vi "Initialize.vi"(0 "DMA FIFO":refnum<k21>="DataSGL7", 5 "instance":u8) -> (4 "subsystem":refnum<class "Single Address Space Collection.lvclass">, 6 "AddressSpace":refnum<class "WaveformAddressSpace.lvclass">)   [LabVIEW 2017, in "WaveformAddressSpace.lvclass"]
uses:
  WaveformAddressSpace.lvclass
  C:/Program Files (x86)/National Instruments/LabVIEW 2017/instr.lib/_niInstr/Instruction Framework/v1/FPGA/Interfaces/Address Space/Address Space.lvclass
  <instrlib>/_niInstr/Instruction Framework/v1/FPGA/Helper Classes/Single Address Space Collection/Single Address Space Collection.lvclass
  Registers.ctl
  WaveformAddressSpace.lvclass/WaveformAddressSpace.ctl
  <vilib>/rvi/DataTransferAndStorage/Container/Common/niFpgaContainerGetUniqueNameForEmu.vi
  <vilib>/rvi/DataTransferAndStorage/Container/Common/niFpgaContainerSetEmuInfo.vi
  <vilib>/rvi/eio/common/nirviEmuReportErrorAndStop.vi
  <vilib>/rvi/LocalResourceManager/LocalResourceManager.xnode
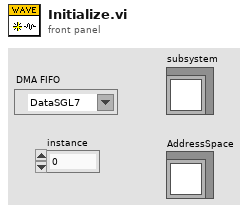
[diagram p1: front panel]
types:
  T1 = typedef "WaveformAddressSpace.lvclass/Registers.ctl" = cluster{"oclk_freq":refnum<k21>, "data_rate":refnum<k21>, "oclk_div":refnum<k21>, "oclk_mult":refnum<k21>, "AcquisitionType":refnum<k21>, "SamplesPerChan":refnum<k21>, "NumberOfChannels":refnum<k21>, "stop":refnum<k21>, "FIFO":refnum<k21>, "FirstRead":refnum<k21>, "ErrorCode":refnum<k21>, "ChannelCount":refnum<k21>, "Finished":refnum<k21>, "DMA_FIFO_Full":refnum<k21>, "ModuleUnderflow":refnum<k21>, "ConfigReadyIRQ":refnum<k21>, "ConfigReadyAck":refnum<k21>, "SynchStartIRQ":refnum<k21>, "SynchStartAck":refnum<k21>, "UnderflowCount":refnum<k21>, "FirstReadReset":refnum<k21>}
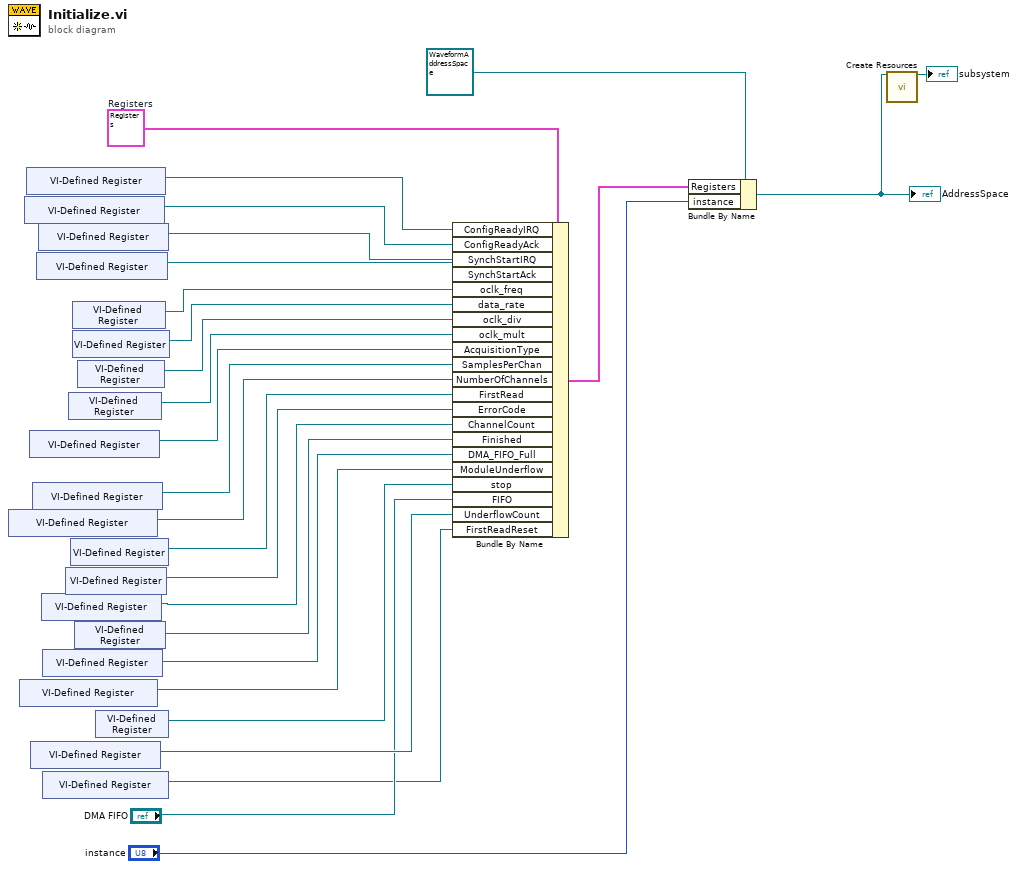
[diagram p0: block diagram]
diagram:
  w12 = T1 {"oclk_freq"="", "data_rate"="", "oclk_div"="", "oclk_mult"="", "AcquisitionType"="", "SamplesPerChan"="", "NumberOfChannels"="", "stop"="", "FIFO"="", "FirstRead"="", "ErrorCode"="", "ChannelCount"="", "Finished"="", "DMA_FIFO_Full"="", "ModuleUnderflow"="", "ConfigReadyIRQ"="Register", "ConfigReadyAck"="Register", "SynchStartIRQ"="Register", "SynchStartAck"="Register", "UnderflowCount"="", "FirstReadReset"="Register"}  # Registers
  n1 = xnode "VI-Defined Register"() -> ("Register Out"=w21:refnum<k21>)
  n2 = xnode "VI-Defined Register"() -> ("Register Out"=w13:refnum<k21>)
  n3 = xnode "VI-Defined Register"() -> ("Register Out"=w7:refnum<k21>)
  n4 = xnode "VI-Defined Register"() -> ("Register Out"=w8:refnum<k21>)
  n5 = xnode "VI-Defined Register"() -> ("Register Out"=w23:refnum<k21>)
  n6 = xnode "VI-Defined Register"() -> ("Register Out"=w4:refnum<k21>)
  n7 = xnode "VI-Defined Register"() -> ("Register Out"=w22:refnum<k21>)
  n8 = xnode "VI-Defined Register"() -> ("Register Out"=w5:refnum<k21>)
  n9 = xnode "VI-Defined Register"() -> ("Register Out"=w6:refnum<k21>)
  n10 = xnode "VI-Defined Register"() -> ("Register Out"=w16:refnum<k21>)
  n11 = xnode "VI-Defined Register"() -> ("Register Out"=w14:refnum<k21>)
  n12 = xnode "VI-Defined Register"() -> ("Register Out"=w1:refnum<k21>)
  n13 = xnode "VI-Defined Register"() -> ("Register Out"=w17:refnum<k21>)
  n14 = xnode "VI-Defined Register"() -> ("Register Out"=w24:refnum<k21>)
  n15 = xnode "VI-Defined Register"() -> ("Register Out"=w19:refnum<k21>)
  n16 = xnode "VI-Defined Register"() -> ("Register Out"=w18:refnum<k21>)
  n17 = xnode "VI-Defined Register"() -> ("Register Out"=w26:refnum<k21>)
  n18 = xnode "VI-Defined Register"() -> ("Register Out"=w15:refnum<k21>)
  n19 = xnode "VI-Defined Register"() -> ("Register Out"=w25:refnum<k21>)
  n20 = xnode "VI-Defined Register"() -> ("Register Out"=w20:refnum<k21>)
  n21 = Bundle By Name(cluster=w12, "ConfigReadyIRQ"=w8, "ConfigReadyAck"=w7, "SynchStartIRQ"=w6, "SynchStartAck"=w5, "oclk_freq"=w18, "data_rate"=w26, "oclk_div"=w25, "oclk_mult"=w24, "AcquisitionType"=w23, "SamplesPerChan"=w22, "NumberOfChannels"=w21, "FirstRead"=w19, "ErrorCode"=w17, "ChannelCount"=w16, "Finished"=w15, "DMA_FIFO_Full"=w14, "ModuleUnderflow"=w13, "stop"=w20, "FIFO"="DMA FIFO", "UnderflowCount"=w4, "FirstReadReset"=w1) -> (w11:T1)
  n22 = Bundle By Name(cluster=refnum<class "WaveformAddressSpace.lvclass"> refnum ("WaveformAddressSpace.lvclass"), "Registers"=w11, "instance"="instance") -> (w10:refnum<class "WaveformAddressSpace.lvclass">)
  "AddressSpace" <- w10
  n23 = call <instrlib>:"Create Resources.vi"("address space"=w10) -> ("single address space collection"=→"subsystem":refnum<class "Single Address Space Collection.lvclass">)  [unwired: 14 in]
